vi "page_2_ctrls.vi"(4 "Error in":errorcluster caption="Error in (no error)", 6 "ctrl ref":refnum<vi>) -> (0 "Error out":errorcluster, 1 "is page?":bool, 2 "ctrls in pages":refnum<vi>[](array[refnum]))   [LabVIEW 2015]
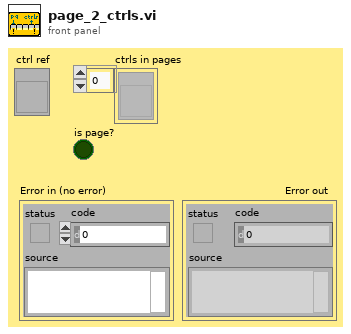
[diagram p1: front panel]
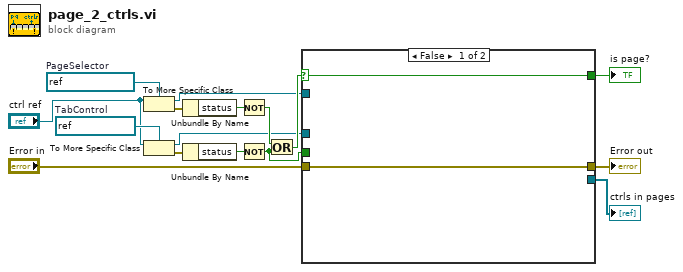
[diagram p0: block diagram]
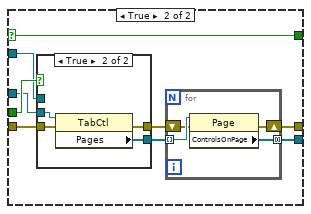
[diagram p2: hidden frame]
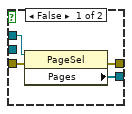
[diagram p3: hidden frame]
diagram:
  w13 = refnum<vi> refnum  # PageSelector
  w14 = refnum<vi> refnum  # TabControl
  n1 = To More Specific Class(target class=w13, reference="ctrl ref") -> (specific class reference=w5:refnum<vi>, error out=w10:errorcluster)  [unwired: 1 in]
  n2 = To More Specific Class(target class=w14, reference="ctrl ref") -> (specific class reference=w6:refnum<vi>, error out=w16:errorcluster)  [unwired: 1 in]
  n3 = Unbundle By Name(w10) -> ("status"=w11:bool)
  n4 = Unbundle By Name(w16) -> ("status"=w15:bool)
  n5 = Not(x=w11) -> (.not. x?=w9:bool)
  n6 = Not(x=w15) -> (.not. x?=w7:bool)
  n7 = Or(x=w9, y=w7) -> (x .or. y?=w8:bool)
  n8 = case shown="False" w8 {
    selector: w8 -> [w18 w22]
    tunnel: w7 -> [_ w27]
    tunnel: w6 -> [_ w26]
    tunnel: w5 -> [_ w25]
    tunnel: [_ w23] -> w4
    tunnel: [w18 w22] -> w3
    tunnel: "Error in" -> [w17 w21]
    tunnel: [w17 w19] -> w1
    frame False {
    }
    frame True {
      n9 = case shown="True" w27 {
        tunnel: w26 -> [_ w35]
        tunnel: w25 -> [w31 _]
        tunnel: [w30 w34] -> w24
        tunnel: w21 -> [w28 w33]
        tunnel: [w29 w32] -> w20
        frame False {
          n10 = property class="PageSel"(reference=w31, error in=w28) -> (error out=w29:errorcluster, "Pages"=w30:refnum<vi>[])  [unwired: 1 out]
        }
        frame True {
          n11 = property class="TabCtl"(reference=w35, error in=w33) -> (error out=w32:errorcluster, "Pages"=w34:refnum<vi>[])  [unwired: 1 out]
        }
      }
      n12 = for {
        tunnel: w24 -> [w39] mode=indexing
        tunnel: [w38] -> w23 mode=concatenating
        shift-right: [w36] -> w19
        shift-left: w20 -> [w37]
        n13 = property class="Page"(reference=w39, error in=w37) -> (error out=w36:errorcluster, "ControlsOnPage"=w38:refnum<vi>[])  [unwired: 1 out]
      }
    }
  }
  "ctrls in pages" <- w4
  "is page?" <- w3
  "Error out" <- w1
